vi "Inside_Entire_Space.vi"(2 "Model       Roll      Pitch       Yaw (deg)":dbl[](array[numeric]) format="%#.2f", 3 "Current Position":dbl[](array[numeric])=[0.0, 200.0, 40.0] format="%.2f", 4 "Envelope":T1=[{"Max"=16000.0, "Min"=14000.0}, {"Max"=1000.0, "Min"=-1000.0}, {"Max"=700.0, "Min"=0.0}] {"Min" format="%#.1f"; "Max" format="%#.1f"}) -> (0 "Error Comments":string, 1 "Box Inside":bool)   [LabVIEW 2011]
uses:
  Box_size.ctl
panel:
  # "X                           Y                          Z"
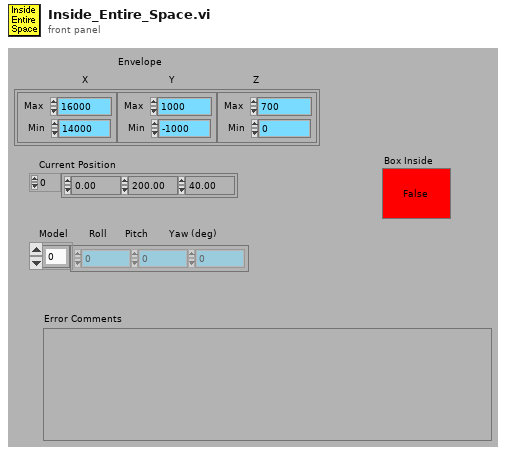
[diagram p1: front panel]
types:
  T1 = typedef "Box_size.ctl" = cluster{"Max":dbl, "Min":dbl}[]
  T2 = enum16{"To Traverse Coordinates", "To User Coordinates"}
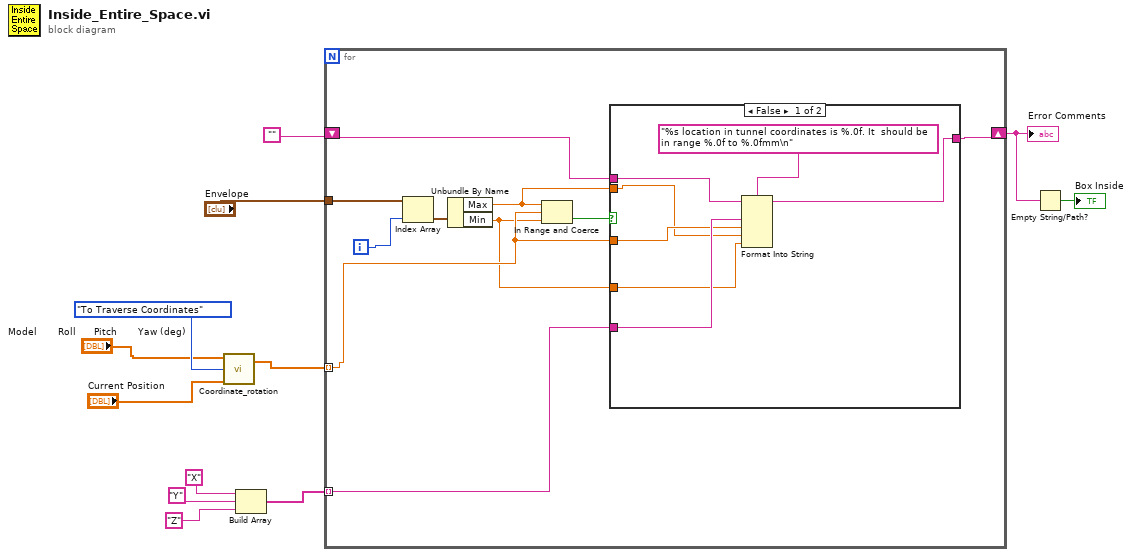
[diagram p0: block diagram]
diagram:
  n1 = call "Coordinate_rotation.vi"("Model       Roll      Pitch       Yaw (deg)"="Model       Roll      Pitch       Yaw (deg)", "Input Position"="Current Position", "Mode"=T2."To Traverse Coordinates") -> ("Output Position"=w4:dbl[])  [unwired: 2 in, 1 out]
  n2 = Build Array("X", "Y", "Z") -> (w8:string[])
  n3 = for {
    shift-left: "" -> [w20]
    shift-right: [w21] -> w5
    tunnel: "Envelope" -> [w22]
    tunnel: w4 -> [w15] mode=indexing
    tunnel: w8 -> [w17] mode=indexing
    i -> [w18]
    n4 = Index Array(array=w22, index=w18) -> (element=w19:cluster{"Max":dbl, "Min":dbl})
    n5 = Unbundle By Name(w19) -> ("Max"=w14:dbl, "Min"=w13:dbl)
    n6 = In Range and Coerce(upper limit=w14, x=w15, lower limit=w13) -> (In Range?=w16:bool)  [unwired: 1 out]
    n7 = case shown="False" w16 {
      tunnel: w20 -> [w28 w30]
      tunnel: [w27 w30] -> w21
      tunnel: w17 -> [w26 _]
      tunnel: w15 -> [w25 _]
      tunnel: w14 -> [w24 _]
      tunnel: w13 -> [w23 _]
      frame False {
        n8 = Format Into String(format string="%s location in tunnel coordinates is %.0f. It  should be in range %.0f to %.0fmm\n" ("Format String"), initial string=w28, w26, w25, w24, w23) -> (resulting string=w27:string)  [unwired: 1 in, 1 out]
      }
      frame True {
      }
    }
  }
  "Error Comments" <- w5
  n9 = Empty String/Path?(string/path=w5) -> (empty?=→"Box Inside":bool)
